vi "习3.5.vi"() -> ()   [LabVIEW 2017]
panel:
  out "数值 2":dbl
  in  "数值":dbl
  out "exp(x)":dbl
  in  "x":dbl
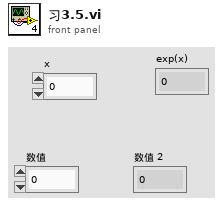
[diagram p1: front panel]
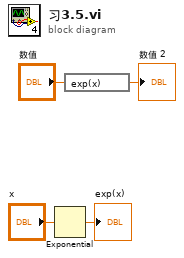
[diagram p0: block diagram]
diagram:
  n1 = Exponential(1:"x") -> (0:→"exp(x)":dbl)
  n2 = expression code="exp(x)"("数值") -> (→"数值 2":dbl)
